vi "Destructor.vi"(8 "error in":errorcluster, 11 "CustomDataType":refnum<class "CustomData.lvclass">) -> (0 "error out":errorcluster)   [LabVIEW 2021, in "ProligentXMLGenerator.lvlib" / "CustomData.lvclass"]
uses:
  CustomData.lvclass
  CustomData.lvclass/CustomData.ctl
  CustomElement/CustomElement.lvclass
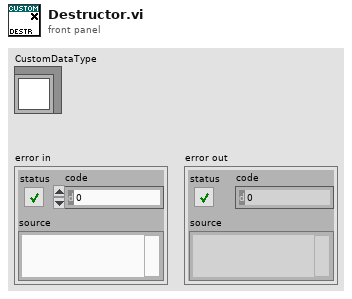
[diagram p1: front panel]
types:
  T1 = typedef "ProligentXMLGenerator.lvlib/CustomData.lvclass/Data.ctl" = cluster{"Name":string, "CustomElements":refnum<class "CustomElement.lvclass">[]}
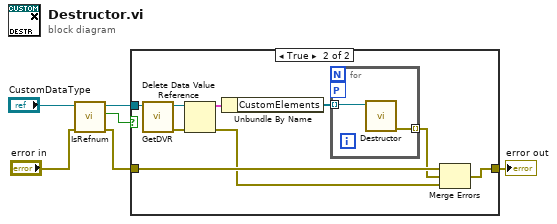
[diagram p0: block diagram]
diagram:
  n1 = call "IsRefnum.vi"("error in"="error in", "CustomDataType in"="CustomDataType") -> ("error out"=w1:errorcluster, "IsRefnum"=w3:bool, "CustomDataType out"=w4:refnum<class "CustomData.lvclass">)  [unwired: 7 in]
  n2 = case shown="True" w3 {
    tunnel: w1 -> [w7 w16]
    tunnel: [w7 w15] -> w6
    tunnel: w4 -> [_ w8]
    frame False {
    }
    frame True {
      n3 = call "GetDVR.vi"("CustomDataType"=w8) -> ("error out"=w13:errorcluster, "DVRReference"=w14:refnum<data-value>)  [unwired: 9 in]
      n4 = Delete Data Value Reference(data value reference=w14, error in=w13) -> (data value=w11:T1, error out=w12:errorcluster)
      n5 = Unbundle By Name(w11) -> ("CustomElements"=w10:refnum<class "CustomElement.lvclass">[])
      n6 = for {
        tunnel: w10 -> [w18] mode=indexing
        tunnel: [w17] -> w9 mode=indexing
        workers-P: _ -> [_]
        n7 = call "Destructor.vi"("CustomElement"=w18) -> ("error out"=w17:errorcluster)  [unwired: 10 in]
      }
      n8 = Merge Errors(w16, w9, w12) -> (w15:errorcluster)
    }
  }
  "error out" <- w6
